vi "Arduino_FlowPump_Controller.vi"(0 "commands":refnum<queue>, 1 "GPIB ADDRESS":string(combo)="1", 2 "DECODER_DATA":refnum<queue>, 3 "measurements":refnum<queue>, 4 "Base Path":path=path "C:/Users/parad/Desktop/MAPI/last") -> ()   [LabVIEW 2021, in "GPIB_UART.lvlib"]
uses:
  GPIB_UART.lvlib
  startup_FSM.ctl
  dc_ps_FSM.ctl
  current_ramp_FSM.ctl
  Agilent_GPIB_FSM.vi
  Arduino_Serial_FSM.vi
  <vilib>/ErrorRing/Error Ring.xnode
panel:
  in  "START":i32
  in  "Next Current Ramp State":bool
  in  "Save As Button":bool
  in  "Stop Button":bool
  out "in_range":bool
  out "Output Current [mA]":i32 min=0 max=1 step=1
  in  "ADJUST":bool
  in  "Knob":ext(knob) scale=0.0..1.0
  out "Arduino UNO Controls":dbl[](graph)
  in  "VOLTAGE":bool
  in  "RESET & CLEAR":bool
  in  "READ ERROR":bool
  in  "Next":bool
  in  "CURRENT LIMIT [mA]":i32=700 min=0 max=1000 step=25
  in  "OUTPUT CHANNEL":enum32{"Channel 1", "Channel 2"}(radio)
  in  "STEP [mA]":i32=25 min=25 max=500 step=25
  in  "CURRENT RAMP":bool
  in  "POWER SUPPLY OUTPUT":bool
  in  "Read Button":bool
  out "SERIAL PORT":string(combo)="COM5"
  in  "Commands":string(combo)
  out "SAMPLE  COUNT":i32
  out "flow meas":dbl caption="FLOW RATE [SLPM]"
  in  "SAMP. FREQ. [HZ]":dbl=1.0 min=1.0 max=2.5 step=0.5
  in  "Clear Buffer":bool
  in  "Connect Button":bool
  out "BAUD":string="9600" caption="BAUD RATE (BIT/S)"
  # "POWER SUPPLY \nCONTROLS"
  # "OUTPUT CURRENT [A]"
  # "A"
  # "mA"
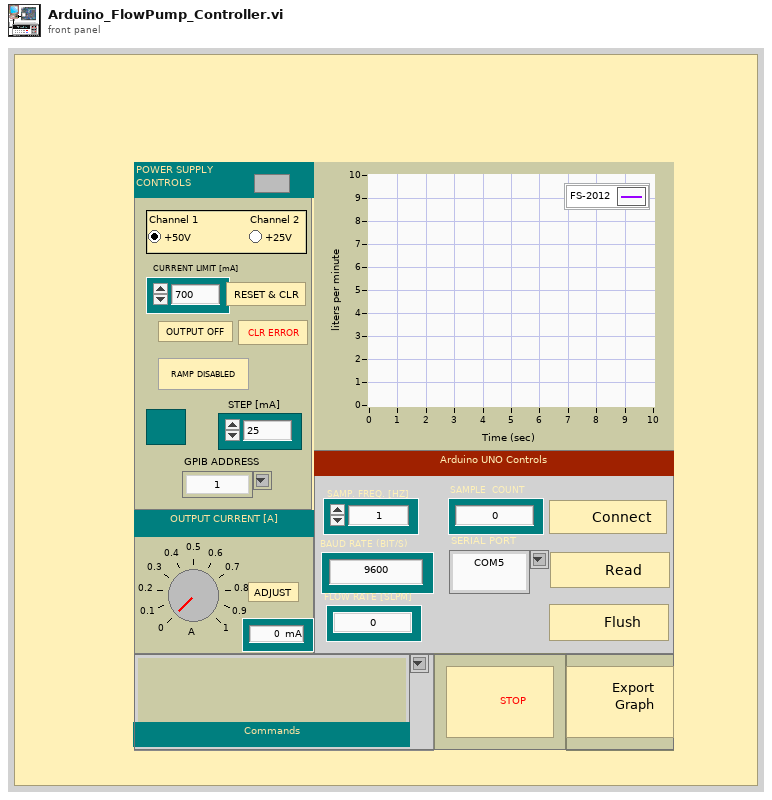
[diagram p1: front panel]
types:
  T1 = typedef "current_ramp_FSM.ctl" = enum16{"STATUS UPDATE", "SHUTDOWN", "INIT", "ERROR", "RAMP SETUP", "RAMP ENABLE", "RAMP DISABLE", "RAMP UP", "RAMP DOWN"}
  T2 = typedef "dc_ps_FSM.ctl" = enum16{"RESET", "SHUTDOWN", "VOLTAGE 12", "VOLTAGE 0", "INIT", "IDLE", "OUTPUT OFF", "OUTPUT ON", "OUT CURR", "SELECT CH", "LIMITS", "ENABLE RAMP", "RAMP UP", "RAMP DOWN", "RAMP STEP", "MEAS", "MEAS?", "ERROR", "READ ERROR", "DISABLE RAMP"}
  T3 = typedef "startup_FSM.ctl" = enum16{"SHUTDOWN", "IDLE", "INIT", "START MEAS", "READ", "STOP MEAS", "CHANGE BAUD", "CHANGE SAMP. FREQ.", "CHANGE PORT", "WRITE", "DISCONNECT", "CONNECT", "OUTPUT OFF", "MEAS_UNIT_L", "MEAS_UNIT_mL", "ERROR", "CLEAR BUFF", "OUTPUT ON"}
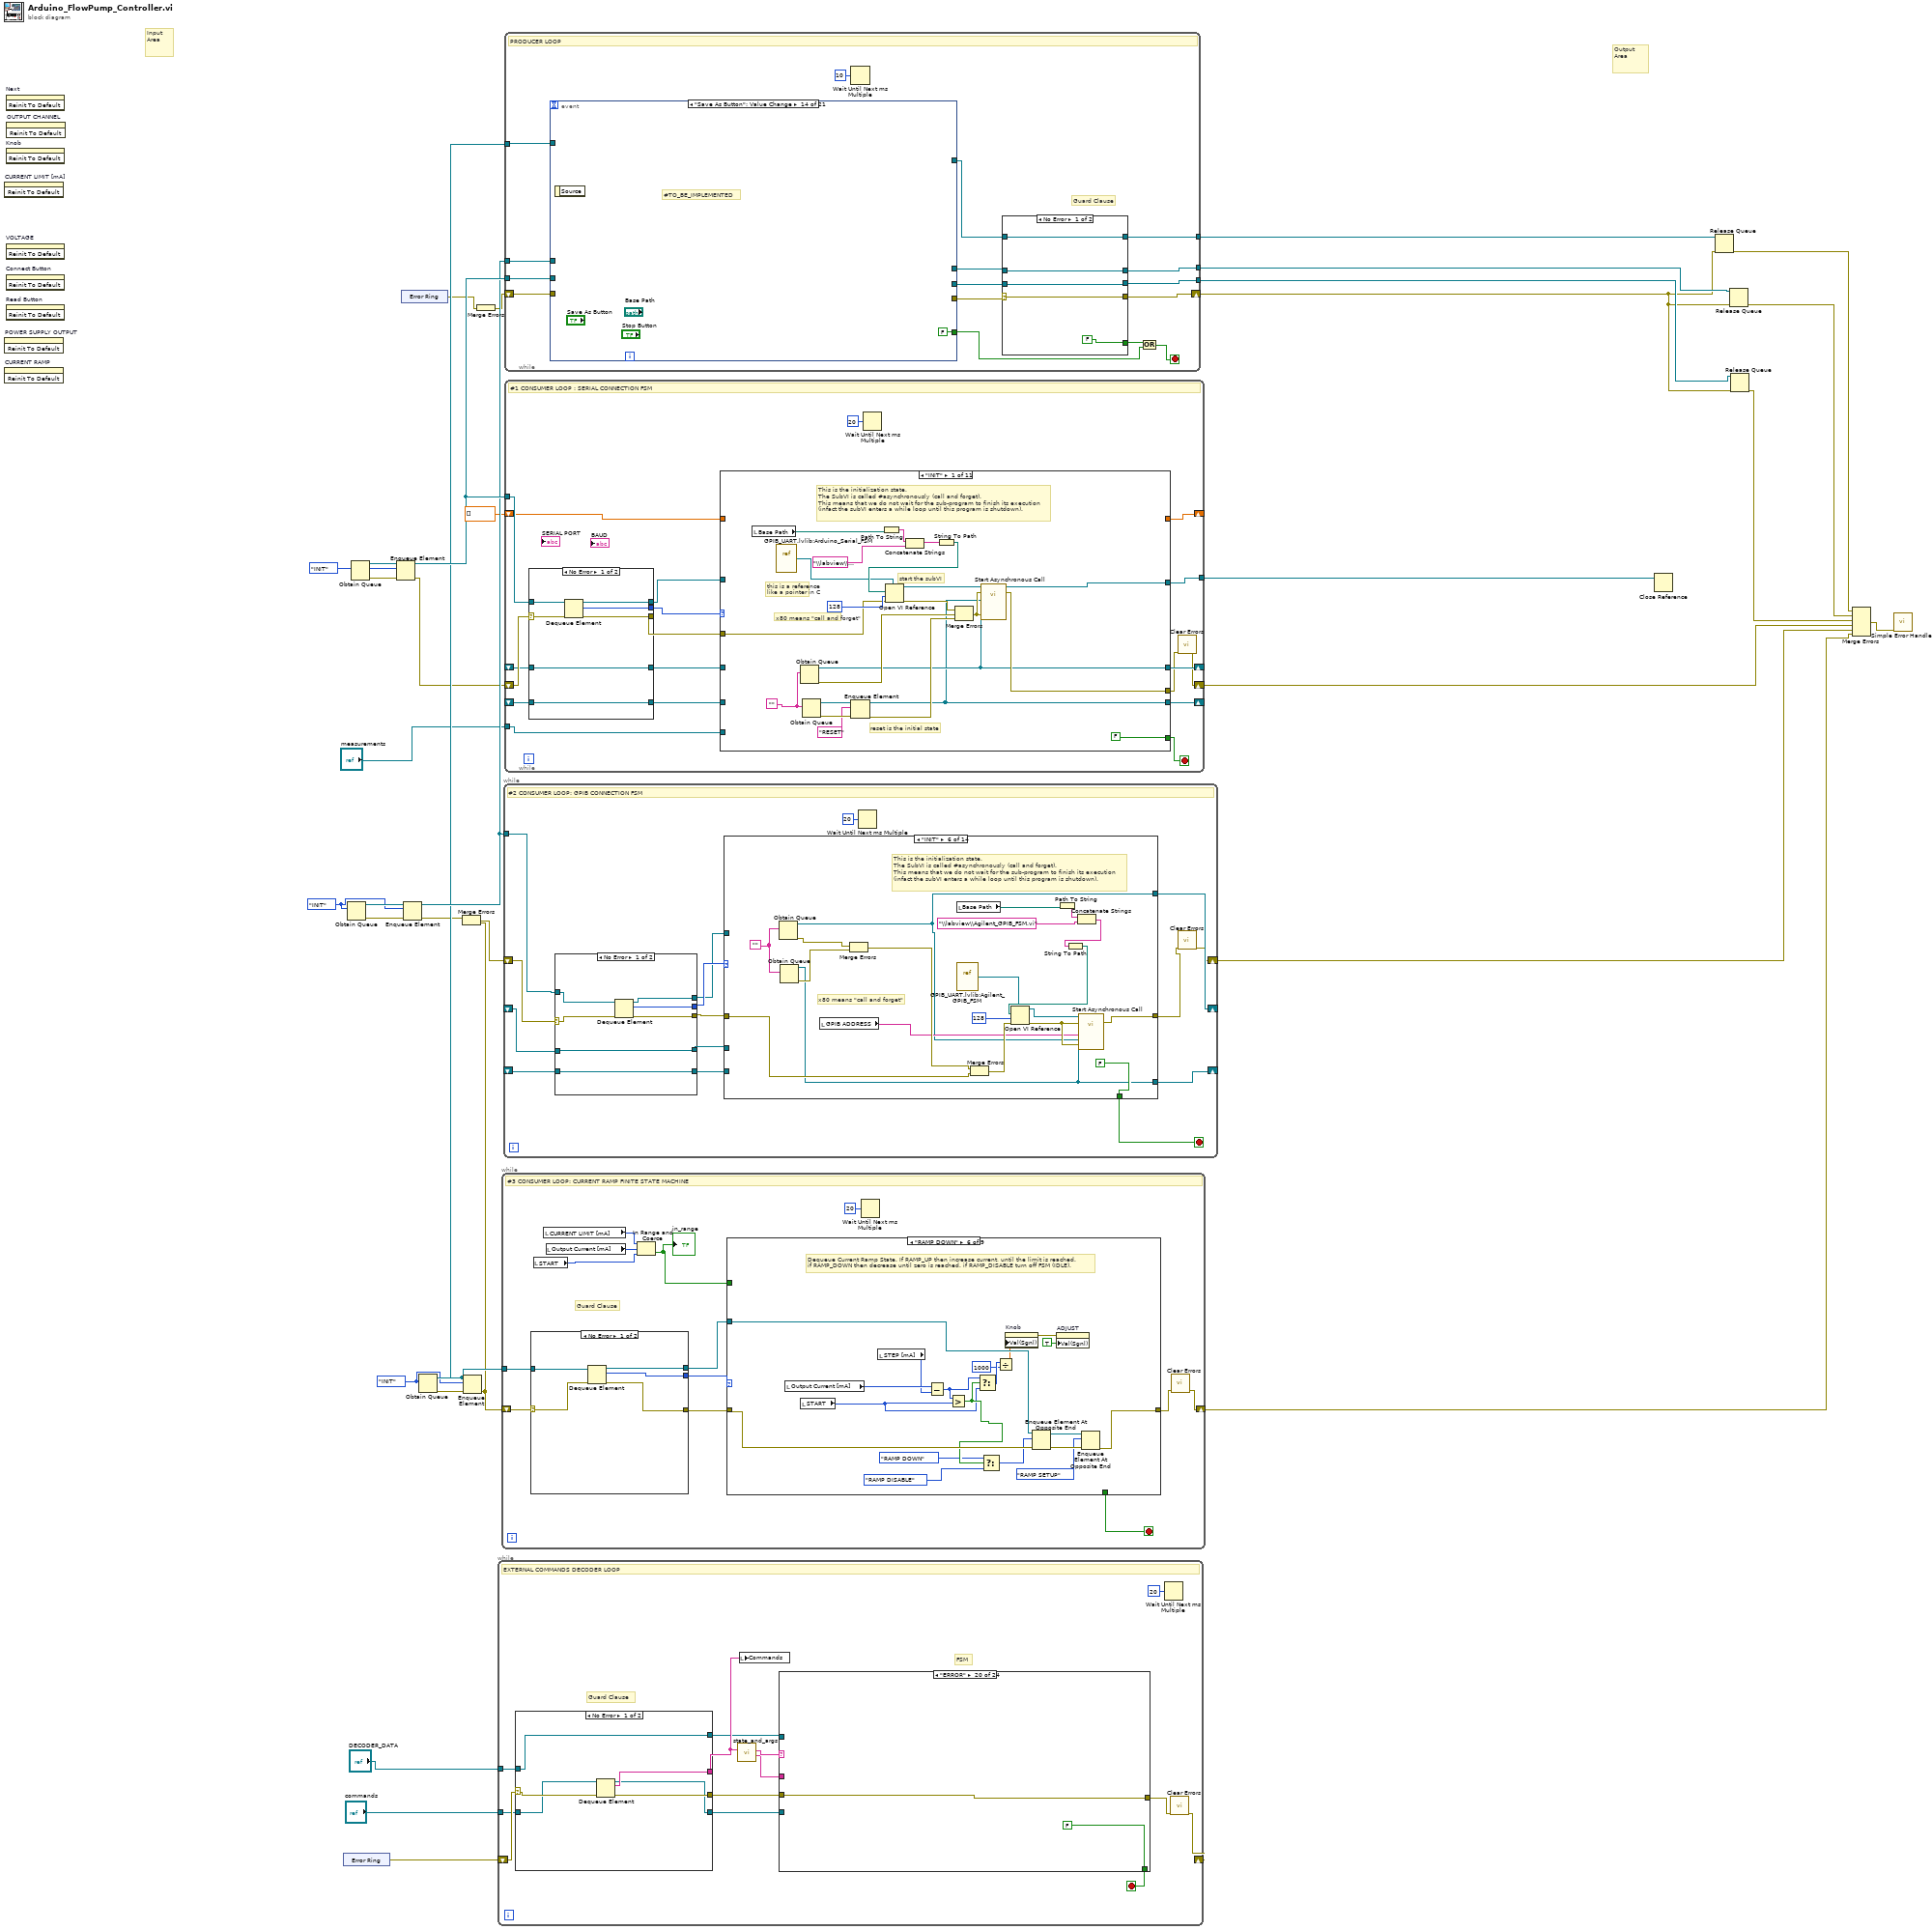
[diagram p0: block diagram]
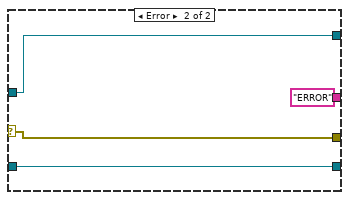
[diagram p2: hidden frame]
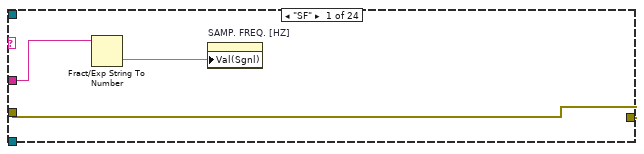
[diagram p3: hidden frame]
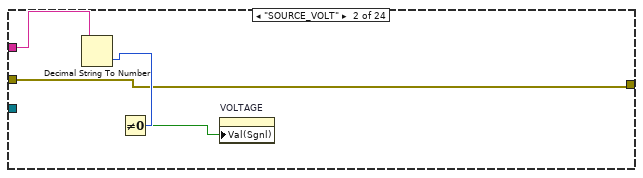
[diagram p4: hidden frame]
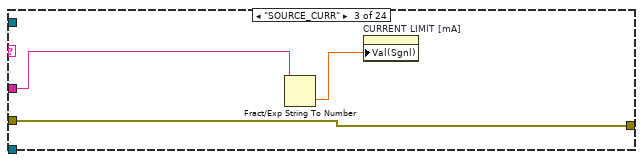
[diagram p5: hidden frame]
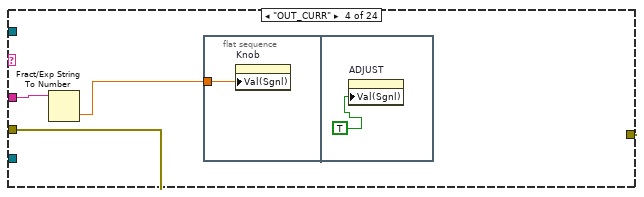
[diagram p6: hidden frame]
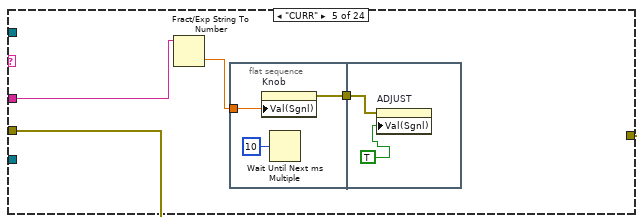
[diagram p7: hidden frame]
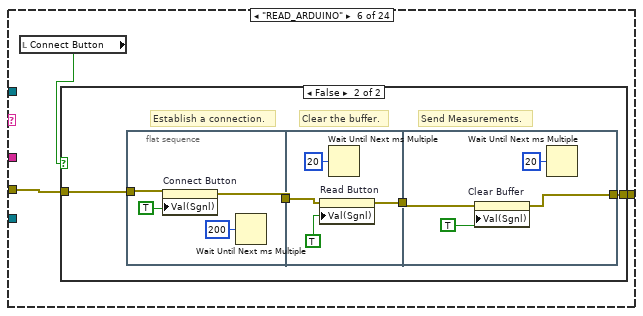
[diagram p8: hidden frame]
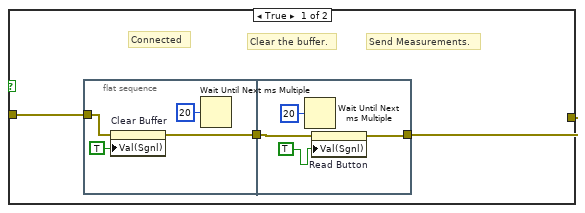
[diagram p9: hidden frame]
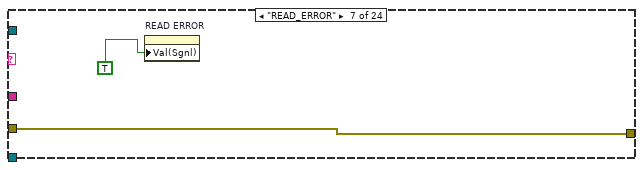
[diagram p10: hidden frame]
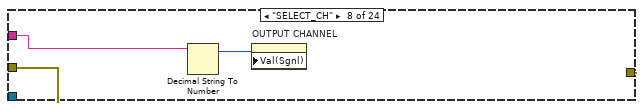
[diagram p11: hidden frame]
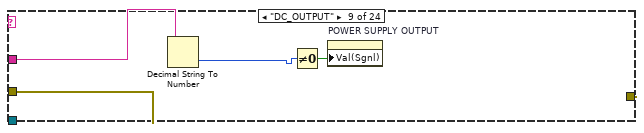
[diagram p12: hidden frame]
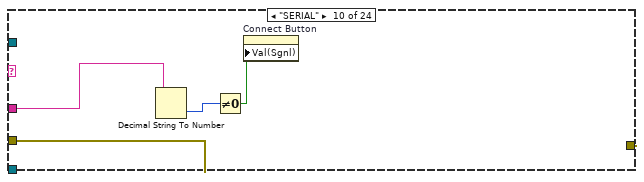
[diagram p13: hidden frame]
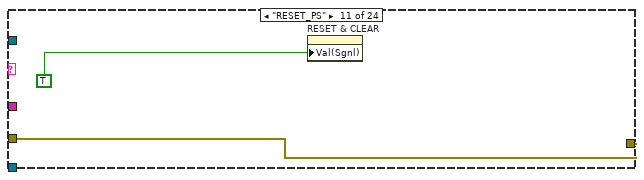
[diagram p14: hidden frame]
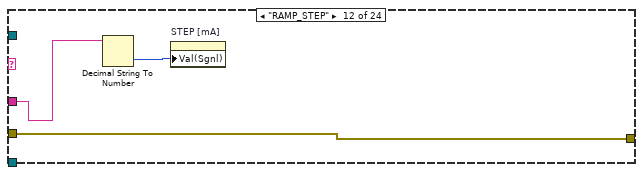
[diagram p15: hidden frame]
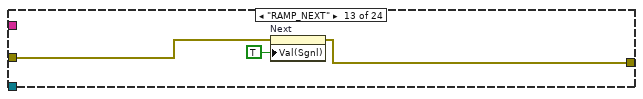
[diagram p16: hidden frame]
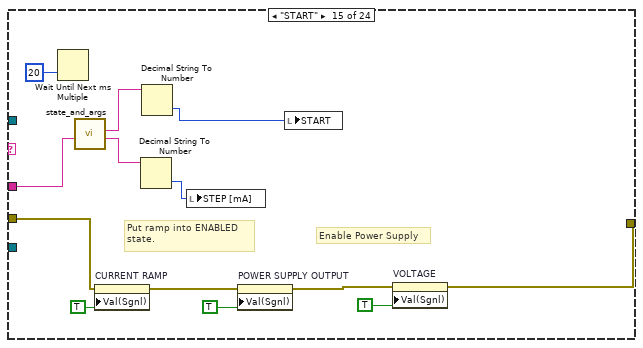
[diagram p18: hidden frame]
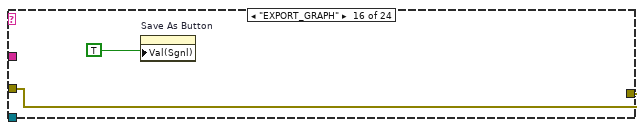
[diagram p19: hidden frame]
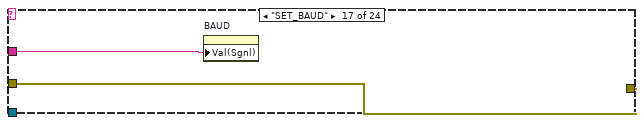
[diagram p20: hidden frame]
diagram:
  w14 = current_ramp_FSM."INIT" ("Enum")
  w29 = dc_ps_FSM."INIT" ("DC Power Supply FSM")
  w30 = startup_FSM."INIT" ("element")
  # "Output\nArea"
  # "Input\nArea"
  n1 = invoke on="CURRENT LIMIT [mA]" class="DigNum (strict)" method="Reinit To Default"() -> ()  [unwired: 3 in, 3 out]
  n2 = invoke on="POWER SUPPLY OUTPUT" class="Bool (strict)" method="Reinit To Default"() -> ()  [unwired: 3 in, 3 out]
  n3 = invoke on="CURRENT RAMP" class="Bool (strict)" method="Reinit To Default"() -> ()  [unwired: 3 in, 3 out]
  n4 = invoke on="Next" class="Bool (strict)" method="Reinit To Default"() -> ()  [unwired: 3 in, 3 out]
  n5 = invoke on="Knob" class="Knob (strict)" method="Reinit To Default"() -> ()  [unwired: 3 in, 3 out]
  n6 = invoke on="VOLTAGE" class="Bool (strict)" method="Reinit To Default"() -> ()  [unwired: 3 in, 3 out]
  n7 = invoke on="Connect Button" class="Bool (strict)" method="Reinit To Default"() -> ()  [unwired: 3 in, 3 out]
  n8 = invoke on="Read Button" class="Bool (strict)" method="Reinit To Default"() -> ()  [unwired: 3 in, 3 out]
  n9 = invoke on="OUTPUT CHANNEL" class="RadioBtnsControl (strict)" method="Reinit To Default"() -> ()  [unwired: 3 in, 3 out]
  n10 = xnode "Error Ring"() -> ("error out"=w15:errorcluster)
  n11 = Obtain Queue(element data type=w29) -> (queue out=w32:refnum<queue>, error out=w31:errorcluster)  [unwired: 4 in, 1 out]
  n12 = Obtain Queue(element data type=w30) -> (queue out=w35:refnum<queue>, error out=w34:errorcluster)  [unwired: 4 in, 1 out]
  n13 = Enqueue Element(queue=w35, element=w30, error in (no error)=w34) -> (queue out=w33:refnum<queue>, error out=w7:errorcluster)  [unwired: 1 in, 1 out]
  n14 = xnode "Error Ring"() -> ("error out"=w11:errorcluster)
  n15 = Enqueue Element(queue=w32, element=w29, error in (no error)=w31) -> (queue out=w28:refnum<queue>, error out=w9:errorcluster)  [unwired: 1 in, 1 out]
  n16 = Obtain Queue(element data type=w14) -> (queue out=w19:refnum<queue>, error out=w18:errorcluster)  [unwired: 4 in, 1 out]
  n17 = Enqueue Element(queue=w19, element=w14, error in (no error)=w18) -> (queue out=w17:refnum<queue>, error out=w8:errorcluster)  [unwired: 1 in, 1 out]
  n18 = Merge Errors(w9, w8) -> (w10:errorcluster)
  n19 = Merge Errors(w11) -> (w12:errorcluster)
  n20 = while {
    shift-right: [w37] -> _
    shift-left: w15 -> [w47]
    tunnel: "commands" -> [w44]
    tunnel: "DECODER_DATA" -> [w39]
    stop <- w45 stop-if-true
    # "FSM"
    # "Guard Clause"
    # "EXTERNAL COMMANDS DECODER LOOP"
    n21 = case shown="No Error" w47 {
      selector: w47 -> [w54 w56]
      tunnel: [w53 "ERROR" ("element")] -> w40
      tunnel: [w52 w56] -> w46
      tunnel: [w49 w57] -> w43
      tunnel: w44 -> [w51 w57]
      tunnel: w39 -> [w50 w55]
      tunnel: [w50 w55] -> w38
      frame No Error {
        n22 = Dequeue Element(queue=w51, error in (no error)=w54) -> (queue out=w49:refnum<queue>, element=w53:string, error out=w52:errorcluster)  [unwired: 1 in, 1 out]
      }
      frame Error {
      }
    }
    n23 = call "state_and_args.vi"("String"=w40) -> ("Arguments"=w41:string, "State"=w42:string)  [unwired: 9 in]
    n24 = local write "Commands"(w40) -> ()
    n25 = case shown="\"ERROR\"" w42 {
      tunnel: w46 -> [w59 w62 w66 w70 w76 w85 w113 w115 w118 w122 w126 w128 w131 w134 w144 w148 w150 w152 w157 w161 w163 w170 w179 w182]
      tunnel: [_ _ _ _ _ _ _ _ _ _ _ _ _ _ _ _ _ _ _ FALSE FALSE _ TRUE _] -> w45
      tunnel: w43 -> [_ _ _ _ _ _ _ _ _ _ _ _ _ _ _ _ _ _ _ _ _ _ _ _]
      tunnel: [w59 w62 w66 w70 w76 w84 w113 w115 w118 w122 w126 w128 w132 w134 w141 w148 w150 w152 w156 w161 w163 w166 w180 w182] -> w36
      tunnel: w41 -> [w60 w63 w67 w69 w75 _ _ w116 w119 w123 _ w129 _ _ w140 _ w151 w153 _ _ _ w169 _ _]
      tunnel: w38 -> [_ _ _ _ _ _ _ _ _ _ _ _ _ _ _ _ _ _ w160 _ _ _ _ _]
      frame "SF" {
        n26 = Fract/Exp String To Number(string=w60) -> (number=w61:dbl)  [unwired: 3 in, 1 out]
        n27 = property on="SAMP. FREQ. [HZ]" class="DigNum (strict)"("Val(Sgnl)"=w61) -> ()  [unwired: 2 in, 2 out]
      }
      frame "SOURCE_VOLT" {
        n28 = Decimal String To Number(string=w63) -> (number=w65:i32)  [unwired: 2 in, 1 out]
        n29 = Not Equal To 0?(x=w65) -> (x != 0?=w64:bool)
        n30 = property on="VOLTAGE" class="Bool (strict)"("Val(Sgnl)"=w64) -> ()  [unwired: 2 in, 2 out]
      }
      frame "SOURCE_CURR" {
        n31 = Fract/Exp String To Number(string=w67) -> (number=w68:dbl)  [unwired: 3 in, 1 out]
        n32 = property on="CURRENT LIMIT [mA]" class="DigNum (strict)"("Val(Sgnl)"=w68) -> ()  [unwired: 2 in, 2 out]
      }
      frame "OUT_CURR" {
        n33 = Fract/Exp String To Number(string=w69) -> (number=w71:dbl)  [unwired: 3 in, 1 out]
        n34 = flat-sequence {
          tunnel: w71 -> [w72]
          frame #0 {
            n35 = property on="Knob" class="Knob (strict)"("Val(Sgnl)"=w72) -> ()  [unwired: 2 in, 2 out]
          }
          frame #1 {
            n36 = property on="ADJUST" class="Bool (strict)"("Val(Sgnl)"=TRUE) -> ()  [unwired: 2 in, 2 out]
          }
        }
      }
      frame "CURR" {
        n37 = Fract/Exp String To Number(string=w75) -> (number=w77:dbl)  [unwired: 3 in, 1 out]
        n38 = flat-sequence {
          tunnel: w77 -> [w80]
          tunnel: [w78] -> w74
          tunnel: w74 -> [w81]
          frame #0 {
            n39 = property on="Knob" class="Knob (strict)"("Val(Sgnl)"=w80) -> (error out=w78:errorcluster)  [unwired: 2 in, 1 out]
            n40 = Wait Until Next ms Multiple(millisecond multiple=u32 10) -> ()  [unwired: 1 out]
          }
          frame #1 {
            n41 = property on="ADJUST" class="Bool (strict)"(error in=w81, "Val(Sgnl)"=TRUE) -> ()  [unwired: 1 in, 2 out]
          }
        }
      }
      frame "READ_ARDUINO" {
        n42 = local read "Connect Button"() -> (w83:bool)
        n43 = case shown="False" w83 {
          tunnel: w85 -> [w86 w100]
          tunnel: [w88 w97] -> w84
          frame True {
            # "Send Measurements."
            # "Clear the buffer."
            # "Connected"
            n44 = flat-sequence {
              tunnel: [w90] -> w87
              tunnel: w86 -> [w91]
              tunnel: [w95] -> w88
              tunnel: w87 -> [w94]
              frame #0 {
                n45 = property on="Clear Buffer" class="Bool (strict)"(error in=w91, "Val(Sgnl)"=TRUE ("Value (Signaling)")) -> (error out=w90:errorcluster)  [unwired: 1 in, 1 out]
                n46 = Wait Until Next ms Multiple(millisecond multiple=u32 20) -> ()  [unwired: 1 out]
              }
              frame #1 {
                n47 = Wait Until Next ms Multiple(millisecond multiple=u32 20) -> ()  [unwired: 1 out]
                n48 = property on="Read Button" class="Bool (strict)"(error in=w94, "Val(Sgnl)"=TRUE ("Value (Signaling)")) -> (error out=w95:errorcluster)  [unwired: 1 in, 1 out]
              }
            }
          }
          frame False {
            # "Send Measurements."
            # "Clear the buffer."
            # "Establish a connection."
            n49 = flat-sequence {
              tunnel: w100 -> [w103]
              tunnel: [w102] -> w99
              tunnel: w99 -> [w107]
              tunnel: [w106] -> w98
              tunnel: w98 -> [w110]
              tunnel: [w109] -> w97
              frame #0 {
                n50 = property on="Connect Button" class="Bool (strict)"(error in=w103, "Val(Sgnl)"=TRUE ("Value (Signaling)")) -> (error out=w102:errorcluster)  [unwired: 1 in, 1 out]
                n51 = Wait Until Next ms Multiple(millisecond multiple=u32 200) -> ()  [unwired: 1 out]
              }
              frame #1 {
                n52 = property on="Read Button" class="Bool (strict)"(error in=w107, "Val(Sgnl)"=TRUE ("Value (Signaling)")) -> (error out=w106:errorcluster)  [unwired: 1 in, 1 out]
                n53 = Wait Until Next ms Multiple(millisecond multiple=u32 20) -> ()  [unwired: 1 out]
              }
              frame #2 {
                n54 = property on="Clear Buffer" class="Bool (strict)"(error in=w110, "Val(Sgnl)"=TRUE ("Value (Signaling)")) -> (error out=w109:errorcluster)  [unwired: 1 in, 1 out]
                n55 = Wait Until Next ms Multiple(millisecond multiple=u32 20) -> ()  [unwired: 1 out]
              }
            }
          }
        }
      }
      frame "READ_ERROR" {
        n56 = property on="READ ERROR" class="Bool (strict)"("Val(Sgnl)"=TRUE) -> ()  [unwired: 2 in, 2 out]
      }
      frame "SELECT_CH" {
        n57 = Decimal String To Number(string=w116) -> (offset past number=w117:i32)  [unwired: 2 in, 1 out]
        n58 = property on="OUTPUT CHANNEL" class="RadioBtnsControl (strict)"("Val(Sgnl)"=w117) -> ()  [unwired: 2 in, 2 out]
      }
      frame "DC_OUTPUT" {
        n59 = Decimal String To Number(string=w119) -> (number=w121:i32)  [unwired: 2 in, 1 out]
        n60 = Not Equal To 0?(x=w121) -> (x != 0?=w120:bool)
        n61 = property on="POWER SUPPLY OUTPUT" class="Bool (strict)"("Val(Sgnl)"=w120) -> ()  [unwired: 2 in, 2 out]
      }
      frame "SERIAL" {
        n62 = Decimal String To Number(string=w123) -> (number=w124:i32)  [unwired: 2 in, 1 out]
        n63 = Not Equal To 0?(x=w124) -> (x != 0?=w125:bool)
        n64 = property on="Connect Button" class="Bool (strict)"("Val(Sgnl)"=w125) -> ()  [unwired: 2 in, 2 out]
      }
      frame "RESET_PS" {
        n65 = property on="RESET & CLEAR" class="Bool"("Val(Sgnl)"=TRUE) -> ()  [unwired: 2 in, 2 out]
      }
      frame "RAMP_STEP" {
        n66 = Decimal String To Number(string=w129) -> (number=w130:i32)  [unwired: 2 in, 1 out]
        n67 = property on="STEP [mA]" class="DigNum (strict)"("Val(Sgnl)"=w130) -> ()  [unwired: 2 in, 2 out]
      }
      frame "RAMP_NEXT" {
        n68 = property on="Next" class="Bool (strict)"(error in=w131, "Val(Sgnl)"=TRUE ("Value (Signaling)")) -> (error out=w132:errorcluster)  [unwired: 1 in, 1 out]
      }
      frame "RAMP_ENABLE" {
      }
      frame "START" {
        # "Enable Power Supply"
        # "Put ramp into ENABLED\nstate."
        n69 = Wait Until Next ms Multiple(millisecond multiple=u32 20) -> ()  [unwired: 1 out]
        n70 = call "state_and_args.vi"("String"=w140) -> ("Arguments"=w137:string, "State"=w138:string)  [unwired: 9 in]
        n71 = property on="CURRENT RAMP" class="Bool (strict)"(error in=w144, "Val(Sgnl)"=TRUE ("Value (Signaling)")) -> (error out=w143:errorcluster)  [unwired: 1 in, 1 out]
        n72 = Decimal String To Number(string=w137) -> (number=w136:i32)  [unwired: 2 in, 1 out]
        n73 = Decimal String To Number(string=w138) -> (number=w139:i32)  [unwired: 2 in, 1 out]
        n74 = local write "STEP [mA]"(w136) -> ()
        n75 = property on="POWER SUPPLY OUTPUT" class="Bool (strict)"(error in=w143, "Val(Sgnl)"=TRUE ("Value (Signaling)")) -> (error out=w142:errorcluster)  [unwired: 1 in, 1 out]
        n76 = local write "START"(w139) -> ()
        n77 = property on="VOLTAGE" class="Bool (strict)"(error in=w142, "Val(Sgnl)"=TRUE ("Value (Signaling)")) -> (error out=w141:errorcluster)  [unwired: 1 in, 1 out]
      }
      frame "EXPORT_GRAPH" {
        n78 = property on="Save As Button" class="Bool (strict)"("Val(Sgnl)"=TRUE ("Value (Signaling)")) -> ()  [unwired: 2 in, 2 out]
      }
      frame "SET_BAUD" {
        n79 = property on="BAUD" class="Str"("Val(Sgnl)"=w151) -> ()  [unwired: 2 in, 2 out]
      }
      frame "READ_ALL" {
        n80 = Decimal String To Number(string=w153) -> (number=w154:i32)  [unwired: 2 in, 1 out]
        n81 = Not Equal To 0?(x=w154) -> (x != 0?=w155:bool)
        n82 = property on="Read Button" class="Bool (strict)"("Val(Sgnl)"=w155) -> ()  [unwired: 2 in, 2 out]
      }
      frame "CURR?" {
        n83 = local read "Output Current [mA]"() -> (w159:i32)
        n84 = Number To Decimal String(number=w159) -> (decimal integer string=w158:string)  [unwired: 1 in]
        n85 = Enqueue Element(queue=w160, element=w158, error in (no error)=w157) -> (error out=w156:errorcluster)  [unwired: 1 in, 2 out]
      }
      frame "ERROR" {
      }
      frame "CLEAR_BUFF" {
        n86 = property on="Clear Buffer" class="Bool (strict)"("Val(Sgnl)"=TRUE ("Value (Signaling)")) -> ()  [unwired: 2 in, 2 out]
      }
      frame "SET_PORT" {
        n87 = local read "Connect Button"() -> (w171:bool)
        n88 = case shown="False" w171 {
          tunnel: w170 -> [w172 w176]
          tunnel: [w172 w175] -> w167
          tunnel: [w173 w174] -> w168
          tunnel: w169 -> [w173 w174]
          frame False {
          }
          frame True {
            n89 = property on="Connect Button" class="Bool (strict)"(error in=w176, "Val(Sgnl)"=FALSE ("Value (Signaling)")) -> (error out=w175:errorcluster)  [unwired: 1 in, 1 out]
          }
        }
        n90 = property on="SERIAL PORT" class="CmbBox"(error in=w167, "Val(Sgnl)"=w168) -> (error out=w166:errorcluster)  [unwired: 1 in, 1 out]
      }
      frame "SHUTDOWN" {
        n91 = property on="Stop Button" class="Bool (strict)"(error in=w179, "Val(Sgnl)"=TRUE) -> (error out=w180:errorcluster)  [unwired: 1 in, 1 out]
      }
      frame "Def", Default {
        # "default: do nothing"
      }
    }
    n92 = Wait Until Next ms Multiple(millisecond multiple=u32 20 ("milliseconds to wait")) -> ()  [unwired: 1 out]
    n93 = call <vilib>:"Clear Errors.vi"("error in (no error)"=w36) -> ("error out"=w37:errorcluster)  [unwired: 5 in, 1 out]
  }
  n94 = while {
    shift-right: [w184] -> w13
    shift-left: w8 -> [w193]
    tunnel: w17 -> [w194]
    stop <- w190 stop-if-true
    # "Guard Clause"
    # "#3 CONSUMER LOOP: CURRENT RAMP FINITE STATE MACHINE"
    n95 = case shown="No Error" w193 {
      selector: w193 -> [w262 w265]
      tunnel: w194 -> [w263 w266]
      tunnel: [w261 w265] -> w192
      tunnel: [w260 w266] -> w191
      tunnel: [w259 current_ramp_FSM."ERROR" ("Enum")] -> w189
      frame No Error {
        n96 = Dequeue Element(queue=w263, error in (no error)=w262) -> (queue out=w260:refnum<queue>, element=w259:T1, error out=w261:errorcluster)  [unwired: 1 in, 1 out]
      }
      frame Error {
      }
    }
    n97 = local read "START"() -> (w183:i32)
    n98 = local read "CURRENT LIMIT [mA]"() -> (w188:i32)
    n99 = local read "Output Current [mA]"() -> (w187:i32)
    n100 = In Range and Coerce(upper limit=w188, x=w187, lower limit=w183) -> (In Range?=w186:bool)  [unwired: 1 out]
    "in_range" <- w186
    n101 = case shown="\"RAMP DOWN\"" w189 {
      tunnel: w192 -> [w199 w202 w210 w211 w214 w234 w254 w258 _]
      tunnel: [w196 w202 w209 w211 w213 w223 w239 w257 _] -> w185
      tunnel: w191 -> [w200 _ w208 _ _ w227 w246 w255 _]
      tunnel: [TRUE FALSE _ _ _ _ _ FALSE _] -> w190
      tunnel: w186 -> [_ _ _ _ _ _ w238 _ _]
      frame "SHUTDOWN" {
        n102 = Preview Queue Element(queue=w200, error in (no error)=w199) -> (queue out=w198:refnum<queue>, error out=w197:errorcluster)  [unwired: 1 in, 2 out]
        n103 = Preview Queue Element(queue=w198, error in (no error)=w197) -> (error out=w196:errorcluster)  [unwired: 1 in, 3 out]
      }
      frame "INIT", Default {
      }
      frame "RAMP ENABLE" {
        n104 = local read "STEP [mA]"() -> (w205:i32)
        n105 = Subtract(x="START", y=w205) -> (x-y=w204:i32)
        n106 = local write "Output Current [mA]"(w204) -> ()
        n107 = Enqueue Element(queue=w208, element=current_ramp_FSM."RAMP UP", error in (no error)=w210) -> (error out=w209:errorcluster)  [unwired: 1 in, 2 out]
      }
      frame "RAMP DISABLE" {
        n108 = property on="CURRENT RAMP" class="Bool (strict)"("Val(Sgnl)"=FALSE ("Value (Signaling)")) -> ()  [unwired: 2 in, 2 out]
      }
      frame "RAMP SETUP" {
        # "IDLE STATE"
        n109 = event shown="[0] \"Next Current Ramp State\": Value Change" {
          selector: _ -> [_]
          dyn-events: _ -> [_]
          timeout: _ -> [_]
          tunnel: [w215] -> w213
          tunnel: w214 -> [w215]
          event "Next Current Ramp State": Value Change {
            n110 = event-data() -> ()  [unwired: 1 in, 1 out]
          }
        }
      }
      frame "RAMP DOWN" {
        # "Dequeue Current Ramp State. If RAMP_UP then increase current, until the limit is reached.\nif RAMP_DOWN then decrease until zero is reached. if RAMP_DISABLE turn off FSM (IDLE)."
        n111 = local read "Output Current [mA]"() -> (w233:i32)
        n112 = local read "START"() -> (w219:i32)
        n113 = local read "STEP [mA]"() -> (w232:i32)
        n114 = Subtract(x=w233, y=w232) -> (x-y=w231:i32)
        n115 = Greater?(x=w231, y=w219) -> (0:w228:bool)
        n116 = Select(t=w231, s=w228, f=w219) -> (s? t:f=w218:i32)
        n117 = Select(t=current_ramp_FSM."RAMP DOWN" ("element"), s=w228, f=current_ramp_FSM."RAMP DISABLE") -> (s? t:f=w226:T1)
        n118 = Divide(x=w218, y=1000) -> (x/y=w216:dbl)
        n119 = property on="Knob" class="Knob (strict)"("Val(Sgnl)"=w216) -> (error out=w230:errorcluster)  [unwired: 2 in, 1 out]
        n120 = Enqueue Element At Opposite End(queue=w227, element=w226, error in (no error)=w234) -> (queue out=w222:refnum<queue>, error out=w221:errorcluster)  [unwired: 1 in, 1 out]
        n121 = property on="ADJUST" class="Bool (strict)"(error in=w230, "Val(Sgnl)"=TRUE ("Value (Signaling)")) -> ()  [unwired: 1 in, 2 out]
        n122 = Enqueue Element At Opposite End(queue=w222, element=current_ramp_FSM."RAMP SETUP", error in (no error)=w221) -> (error out=w223:errorcluster)  [unwired: 1 in, 2 out]
      }
      frame "RAMP UP" {
        # "Dequeue Current Ramp State. If RAMP_UP then increase current, until the limit is reached."
        n123 = local read "Output Current [mA]"() -> (w253:i32)
        n124 = local read "CURRENT LIMIT [mA]"() -> (w249:i32)
        n125 = local read "STEP [mA]"() -> (w252:i32)
        n126 = Add(x=w253, y=w252) -> (x+y=w250:i32)
        n127 = Less?(x=w250, y=w249) -> (x < y?=w251:bool)
        n128 = Select(t=w250, s=w251, f=w249) -> (s? t:f=w237:i32)
        n129 = Select(t=current_ramp_FSM."RAMP UP" ("element"), s=w238, f=current_ramp_FSM."RAMP DOWN") -> (s? t:f=w243:T1)
        n130 = Divide(x=w237, y=1000) -> (x/y=w235:dbl)
        n131 = property on="Knob" class="Knob (strict)"("Val(Sgnl)"=w235) -> (error out=w248:errorcluster)  [unwired: 2 in, 1 out]
        n132 = Enqueue Element At Opposite End(queue=w246, element=w243, error in (no error)=w254) -> (queue out=w242:refnum<queue>, error out=w241:errorcluster)  [unwired: 1 in, 1 out]
        n133 = Enqueue Element At Opposite End(queue=w242, element=current_ramp_FSM."RAMP SETUP", error in (no error)=w241) -> (error out=w239:errorcluster)  [unwired: 1 in, 2 out]
        n134 = property on="ADJUST" class="Bool (strict)"(error in=w248, "Val(Sgnl)"=TRUE ("Value (Signaling)")) -> ()  [unwired: 1 in, 2 out]
      }
      frame "ERROR" {
        n135 = Preview Queue Element(queue=w255, error in (no error)=w258) -> (error out=w257:errorcluster)  [unwired: 1 in, 3 out]
      }
      frame "STATUS UPDATE" {
      }
    }
    n136 = Wait Until Next ms Multiple(millisecond multiple=u32 20) -> ()  [unwired: 1 out]
    n137 = call <vilib>:"Clear Errors.vi"("error in (no error)"=w185) -> ("error out"=w184:errorcluster)  [unwired: 5 in, 1 out]
  }
  n138 = while {
    tunnel: w28 -> [w280]
    shift-right: [w268] -> w22
    shift-left: w10 -> [w281]
    shift-right: [w271] -> _
    shift-left: _ -> [w270]
    shift-right: [w272] -> _
    shift-left: _ -> [w273]
    stop <- w276 stop-if-true
    # "#2 CONSUMER LOOP: GPIB CONNECTION FSM"
    n139 = case shown="No Error" w281 {
      selector: w281 -> [w418 w422]
      tunnel: w280 -> [w419 w423]
      tunnel: [w417 dc_ps_FSM."ERROR" ("DC Power Supply FSM")] -> w279
      tunnel: [w416 w423] -> w278
      tunnel: [w415 w422] -> w277
      tunnel: w273 -> [w414 w420]
      tunnel: [w414 w420] -> w274
      tunnel: [w413 w421] -> w269
      tunnel: w270 -> [w413 w421]
      frame No Error {
        n140 = Dequeue Element(queue=w419, error in (no error)=w418) -> (queue out=w416:refnum<queue>, element=w417:T2, error out=w415:errorcluster)  [unwired: 1 in, 1 out]
      }
      frame Error {
      }
    }
    n141 = case shown="\"INIT\"" w279 {
      tunnel: w278 -> [_ _ _ _ _ _ w354 _ _ _ _ _ _ _]
      tunnel: w277 -> [w286 w293 w304 w309 w332 w340 w353 w378 w385 w391 w396 w403 w408 w412]
      tunnel: [w285 w291 w299 w308 w327 w350 w355 w380 w385 w389 w395 w402 w407 w412] -> w267
      tunnel: w274 -> [w282 w288 w296 w305 w324 _ w359 w377 w384 w387 w394 w399 w404 w410]
      tunnel: [_ _ _ _ _ FALSE TRUE FALSE _ _ _ _ _ _] -> w276
      tunnel: [w282 w288 w296 w305 w324 w333 w359 w375 w384 w387 w394 w399 w404 w410] -> w272
      tunnel: [w283 w289 w295 w306 w325 w334 w356 w374 w383 w386 w392 w398 w405 w411] -> w271
      tunnel: w269 -> [w284 w290 w297 w307 w326 _ w360 w376 w383 w388 w393 w400 w406 w411]
      frame "OUTPUT OFF" {
        # "Sends a command to the Finite State Machine to turn off its output"
        n142 = Enqueue Element(queue=w284, element="OUTPUT OFF", error in (no error)=w286) -> (queue out=w283:refnum<queue>, error out=w285:errorcluster)  [unwired: 1 in, 1 out]
      }
      frame "OUTPUT ON" {
        # "Sends a command to the Finite State Machine to turn off its output"
        n143 = Enqueue Element(queue=w290, element="OUTPUT ON", error in (no error)=w293) -> (queue out=w289:refnum<queue>, error out=w291:errorcluster)  [unwired: 1 in, 1 out]
      }
      frame "OUT CURR" {
        # "Sends a command to the Finite State Machine to change the output current"
        n144 = local read "Knob"() -> (w294:ext)
        n145 = Number To Fractional String(use system decimal point (T)=FALSE, number=w294, precision (6)=i16 4) -> (F-format string=w303:string)  [unwired: 1 in]
        n146 = Concatenate Strings("CURR " ("element"), w303) -> (w300:string)
        n147 = Enqueue Element(queue=w297, element=w300, error in (no error)=w304) -> (queue out=w295:refnum<queue>, error out=w299:errorcluster)  [unwired: 1 in, 1 out]
      }
      frame "SELECT CH" {
        # "Sends a command to the Finite State Machine to change the output Channel (either 25 or 50V)"
        n148 = case shown="\"Channel 2\", Default" "OUTPUT CHANNEL" {
          tunnel: w309 -> [w315 w320]
          tunnel: [w313 w318] -> w308
          tunnel: w307 -> [w312 w316]
          tunnel: [w311 w317] -> w306
          frame "Channel 1" {
            n149 = Enqueue Element(queue=w312, element="VOLT:RANG P50V", error in (no error)=w315) -> (queue out=w311:refnum<queue>, error out=w313:errorcluster)  [unwired: 1 in, 1 out]
          }
          frame "Channel 2", Default {
            n150 = Enqueue Element(queue=w316, element="VOLT:RANG P25V", error in (no error)=w320) -> (queue out=w317:refnum<queue>, error out=w318:errorcluster)  [unwired: 1 in, 1 out]
          }
        }
      }
      frame "LIMITS" {
        # "Sends a command to the Finite State Machine to change the current limit"
        n151 = Divide(x="CURRENT LIMIT [mA]", y=1000.0) -> (x/y=w321:dbl)
        n152 = Number To Fractional String(number=w321, precision (6)=i16 4) -> (F-format string=w329:string)  [unwired: 2 in]
        n153 = Concatenate Strings("CURR:PROT " ("element"), w329) -> (w331:string)
        n154 = Enqueue Element(queue=w326, element=w331, error in (no error)=w332) -> (queue out=w325:refnum<queue>, error out=w327:errorcluster)  [unwired: 1 in, 1 out]
      }
      frame "INIT" {
        w344 = ""
        # "x80 means \"call and forget\""
        # "This is the initialization state.\nThe SubVI is called #asynchronously (call and forget).\nThis means that we do not wait for the sub-program to finish its execution\n(infact the subVI enters a while loop until this program is shutdown)."
        n155 = Obtain Queue(element data type=w344) -> (queue out=w333:refnum<queue>, error out=w343:errorcluster)  [unwired: 4 in, 1 out]
        n156 = Obtain Queue(element data type=w344) -> (queue out=w334:refnum<queue>, error out=w342:errorcluster)  [unwired: 4 in, 1 out]
        n157 = local read "GPIB ADDRESS"() -> (w337:string)
        n158 = Merge Errors(w343, w342) -> (w341:errorcluster)
        n159 = local read "Base Path"() -> (w349:path)
        n160 = vi-ref "GPIB_UART.lvlib:Agilent_GPIB_FSM.vi"() -> (w336:refnum<vi>)
        n161 = Merge Errors(w341, w340) -> (w339:errorcluster)
        n162 = Path To String(path=w349) -> (string=w348:string)
        n163 = Concatenate Strings(w348, "\\labview\\Agilent_GPIB_FSM.vi" ("string")) -> (w346:string)
        n164 = String To Path(string=w346) -> (path=w345:path)
        n165 = Open VI Reference(type specifier VI Refnum (for type only)=w336, vi path=w345, options=128, error in (no error)=w339) -> (vi reference=w335:refnum<vi>, error out=w338:errorcluster)  [unwired: 2 in]
        n166 = call-by-ref "Start Asynchronous Call"(reference=w335, error in=w338, "error in"=w338, "MEAS"=w333, "GPIB"=w337, "commands"=w334) -> (error out=w350:errorcluster)  [unwired: 7 in, 1 out]
      }
      frame "SHUTDOWN" {
        # "Shutdown gracefully."
        n167 = Flush Queue(queue=w354, error in (no error)=w353) -> ()  [unwired: 3 out]
        n168 = flat-sequence {
          tunnel: w360 -> [w367]
          tunnel: w353 -> [w365]
          tunnel: [w364] -> w358
          tunnel: [w363] -> w357
          tunnel: w358 -> [w373]
          tunnel: w357 -> [w371]
          tunnel: [w370] -> w356
          tunnel: [w369] -> w355
          frame #0 {
            n169 = Wait Until Next ms Multiple(millisecond multiple=u32 100) -> ()  [unwired: 1 out]
            n170 = Enqueue Element(queue=w367, element="RESET", error in (no error)=w365) -> (queue out=w364:refnum<queue>, error out=w363:errorcluster)  [unwired: 1 in, 1 out]
          }
          frame #1 {
            n171 = Wait Until Next ms Multiple(millisecond multiple=u32 100) -> ()  [unwired: 1 out]
            n172 = Enqueue Element(queue=w373, element="SHUTDOWN", error in (no error)=w371) -> (queue out=w370:refnum<queue>, error out=w369:errorcluster)  [unwired: 1 in, 1 out]
          }
        }
      }
      frame "ERROR" {
        # "Release (Destroy) Queues"
        n173 = Preview Queue Element(queue=w376, error in (no error)=w378) -> (queue out=w374:refnum<queue>, error out=w382:errorcluster)  [unwired: 1 in, 2 out]
        n174 = Preview Queue Element(queue=w377, error in (no error)=w378) -> (queue out=w375:refnum<queue>, error out=w381:errorcluster)  [unwired: 1 in, 2 out]
        n175 = Merge Errors(w382, w381) -> (w380:errorcluster)
      }
      frame "IDLE", Default {
      }
      frame "READ ERROR" {
        # "Sends a command to the Finite State Machine to clear any error."
        n176 = Enqueue Element(queue=w388, element="READ:ERROR", error in (no error)=w391) -> (queue out=w386:refnum<queue>, error out=w389:errorcluster)  [unwired: 1 in, 1 out]
      }
      frame "RESET" {
        # "Sends a command to the Finite State Machine to reset the power supply to the settings as when it was turned on the first time."
        n177 = Enqueue Element(queue=w393, element="RESET", error in (no error)=w396) -> (queue out=w392:refnum<queue>, error out=w395:errorcluster)  [unwired: 1 in, 1 out]
      }
      frame "VOLTAGE 12" {
        # "Sends a command to the Finite State Machine to output a voltage that can power the air pump."
        n178 = Enqueue Element(queue=w400, element="VOLT 12", error in (no error)=w403) -> (queue out=w398:refnum<queue>, error out=w402:errorcluster)  [unwired: 1 in, 1 out]
      }
      frame "VOLTAGE 0" {
        # "Sends a command to the Finite State Machine to stop outputting a voltage that can power the air pump."
        n179 = Enqueue Element(queue=w406, element="VOLT 0", error in (no error)=w408) -> (queue out=w405:refnum<queue>, error out=w407:errorcluster)  [unwired: 1 in, 1 out]
      }
      frame "RAMP STEP" {
      }
    }
    n180 = Wait Until Next ms Multiple(millisecond multiple=u32 20) -> ()  [unwired: 1 out]
    n181 = call <vilib>:"Clear Errors.vi"("error in (no error)"=w267) -> ("error out"=w268:errorcluster)  [unwired: 5 in, 1 out]
  }
  n182 = while {
    tunnel: w33 -> [w440]
    shift-right: [w438] -> w5
    shift-left: w12 -> [w439]
    tunnel: w28 -> [w437]
    tunnel: [w436] -> w27
    tunnel: [w435] -> w26
    tunnel: w17 -> [w430]
    tunnel: [w425] -> w6
    stop <- w427 stop-if-true
    # "Guard Clause"
    # "PRODUCER LOOP"
    n183 = event shown="[13] \"Save As Button\": Value Change" {
      selector: _ -> [_ _ _ _ _ _ _ _ _ _ _ _ _ _ _ _ _ _ _ _ _]
      dyn-events: _ -> [_ _ _ _ _ _ _ _ _ _ _ _ _ _ _ _ _ _ _ _ _]
      timeout: _ -> [_ _ _ _ _ _ _ _ _ _ _ _ _ _ _ _ _ _ _ _ _]
      tunnel: w440 -> [w462 _ w476 _ _ w490 _ _ _ _ w551 _ _ _ w598 _ w644 w650 _ _ w678]
      tunnel: w439 -> [w460 _ w470 w480 _ w488 w510 w520 w530 w540 w550 w570 w587 _ w600 w629 w642 w648 w654 w668 w675]
      tunnel: [w458 _ w468 w478 _ w485 w509 w518 w528 w538 w547 w569 w579 _ w591 w628 w636 w646 w652 w662 w676] -> w434
      tunnel: [_ _ w472 _ _ w489 _ _ _ _ _ _ _ _ w593 _ w639 w647 _ _ w677] -> w432
      tunnel: w437 -> [_ _ _ _ _ _ w516 w526 w536 w543 w549 _ w589 _ w603 w634 _ _ w660 w673 _]
      tunnel: [_ _ _ _ _ _ w512 w524 w534 w542 _ _ w588 _ w592 _ _ _ w656 w671 _] -> w433
      tunnel: w430 -> [_ _ _ _ _ _ _ _ _ _ w548 _ _ _ w599 _ _ _ _ _ _]
      tunnel: [FALSE FALSE FALSE FALSE FALSE FALSE FALSE FALSE FALSE FALSE FALSE FALSE FALSE FALSE TRUE FALSE FALSE FALSE FALSE FALSE FALSE] -> w428
      tunnel: [_ _ _ _ _ _ _ _ _ _ _ _ _ _ w594 _ _ _ _ _ _] -> w426
      event "BAUD": Value Change {
        # "Baud Rate Value Changed. Use #1 Consumer Loop to update \nthe Serial Connection Finite State Machine (FSM) status. \nThen, go back to idle state (wait for next event to happen).\nAlso write on the datalog that this event has happened (same for every event case)."
        n184 = event-data() -> ()  [unwired: 1 in, 1 out]
        n185 = Enqueue Element(queue=w462, element=startup_FSM."CHANGE BAUD", error in (no error)=w460) -> (error out=w458:errorcluster)  [unwired: 1 in, 2 out]
      }
      event "Knob": Value Change {
        n186 = event-data() -> ("NewVal"=w464:ext)  [unwired: 1 in]
        n187 = Multiply(x=w464, y=ext 1000.0) -> (x*y=→"Output Current [mA]":ext)
      }
      event "SAMP. FREQ. [HZ]": Value Change {
        # "Sampling Frequency Value Changed. Use #1 Consumer Loop to update \nthe Serial Connection Finite State Machine (FSM) status."
        n188 = event-data() -> ()  [unwired: 1 in, 1 out]
        n189 = Enqueue Element(queue=w476, element=startup_FSM."CHANGE SAMP. FREQ.", error in (no error)=w470) -> (queue out=w474:refnum<queue>, error out=w473:errorcluster)  [unwired: 1 in, 1 out]
        n190 = Enqueue Element(queue=w474, element=startup_FSM."IDLE", error in (no error)=w473) -> (queue out=w472:refnum<queue>, error out=w469:errorcluster)  [unwired: 1 in, 1 out]
        n191 = Merge Errors(w469) -> (w468:errorcluster)
      }
      event "Commands": Value Change {
        # "A new command was enqueued via the front panel. The EXTERNAL COMMANDS DECODER Loop decodes\nthe instruction.\nAlso write on the datalog that this event has happened (same for every event case)."
        n192 = event-data() -> ()  [unwired: 1 in, 1 out]
        n193 = local read "commands"() -> (w482:refnum<queue>)
        n194 = Enqueue Element(queue=w482, element="Commands", error in (no error)=w480) -> (error out=w479:errorcluster)  [unwired: 1 in, 2 out]
        n195 = Merge Errors(w479) -> (w478:errorcluster)
      }
      event "GPIB ADDRESS": Value Change {
        # "#TO_BE_IMPLEMENTED"
        n196 = event-data() -> ()  [unwired: 1 in, 6 out]
      }
      event "Connect Button": Value Change {
        # "Connect Button Value Changed. Either Connect or Disconnect from Arduino.\nThis depends on the value (either true or false) of the connect button)."
        n197 = event-data() -> ("NewVal"=w487:bool)  [unwired: 1 in]
        n198 = case shown="False" w487 {
          tunnel: w490 -> [w498 w506]
          tunnel: [w494 w502] -> w486
          tunnel: [w493 w501] -> w489
          tunnel: w488 -> [w491 w499]
          frame False {
            n199 = Enqueue Element(queue=w498, element=startup_FSM."DISCONNECT", error in (no error)=w491) -> (queue out=w496:refnum<queue>, error out=w495:errorcluster)  [unwired: 1 in, 1 out]
            n200 = Enqueue Element(queue=w496, element=startup_FSM."IDLE", error in (no error)=w495) -> (queue out=w493:refnum<queue>, error out=w494:errorcluster)  [unwired: 1 in, 1 out]
          }
          frame True {
            n201 = Enqueue Element(queue=w506, element=startup_FSM."CONNECT", error in (no error)=w499) -> (queue out=w504:refnum<queue>, error out=w503:errorcluster)  [unwired: 1 in, 1 out]
            n202 = Enqueue Element(queue=w504, element=startup_FSM."IDLE", error in (no error)=w503) -> (queue out=w501:refnum<queue>, error out=w502:errorcluster)  [unwired: 1 in, 1 out]
          }
        }
        n203 = Merge Errors(w486) -> (w485:errorcluster)
      }
      event "STEP [mA]": Value Change {
        # "Current Ramp Step Value Changed. Use the #4 Consumer Loop \nto update the Current Ramp Finite  State Machine status."
        n204 = event-data() -> ()  [unwired: 1 in, 1 out]
        n205 = Enqueue Element(queue=w516, element=dc_ps_FSM."RAMP STEP", error in (no error)=w510) -> (queue out=w514:refnum<queue>, error out=w511:errorcluster)  [unwired: 1 in, 1 out]
        n206 = Enqueue Element(queue=w514, element=dc_ps_FSM."IDLE", error in (no error)=w511) -> (queue out=w512:refnum<queue>, error out=w508:errorcluster)  [unwired: 1 in, 1 out]
        n207 = Merge Errors(w508) -> (w509:errorcluster)
      }
      event "OUTPUT CHANNEL": Value Change {
        # "Changed the Power Supply Output Channel (either 25V or 50V)"
        n208 = event-data() -> ()  [unwired: 1 in, 1 out]
        n209 = Enqueue Element(queue=w526, element=dc_ps_FSM."SELECT CH", error in (no error)=w520) -> (queue out=w525:refnum<queue>, error out=w523:errorcluster)  [unwired: 1 in, 1 out]
        n210 = Enqueue Element(queue=w525, element=dc_ps_FSM."IDLE", error in (no error)=w523) -> (queue out=w524:refnum<queue>, error out=w519:errorcluster)  [unwired: 1 in, 1 out]
        n211 = Merge Errors(w519) -> (w518:errorcluster)
      }
      event "READ ERROR": Value Change {
        # "When a Power Supply Error (like requiring to output 30V using a 25V output channel) it is required to Read (clear) the error to continue to use the instrument."
        n212 = event-data() -> ()  [unwired: 1 in, 1 out]
        n213 = Enqueue Element(queue=w536, element=dc_ps_FSM."READ ERROR", error in (no error)=w530) -> (queue out=w535:refnum<queue>, error out=w533:errorcluster)  [unwired: 1 in, 1 out]
        n214 = Enqueue Element(queue=w535, element=dc_ps_FSM."IDLE", error in (no error)=w533) -> (queue out=w534:refnum<queue>, error out=w529:errorcluster)  [unwired: 1 in, 1 out]
        n215 = Merge Errors(w529) -> (w528:errorcluster)
      }
      event "RESET & CLEAR": Value Change {
        n216 = event-data() -> ()  [unwired: 1 in, 1 out]
        n217 = Enqueue Element(queue=w543, element=dc_ps_FSM."RESET", error in (no error)=w540) -> (queue out=w542:refnum<queue>, error out=w539:errorcluster)  [unwired: 1 in, 1 out]
        n218 = Merge Errors(w539) -> (w538:errorcluster)
      }
      event "CURRENT RAMP": Value Change {
        n219 = event-data() -> ("NewVal"=w552:bool)  [unwired: 1 in]
        n220 = case shown="True" w552 {
          tunnel: w551 -> [_ _]
          tunnel: w550 -> [_ w566]
          tunnel: [_ w562] -> w545
          tunnel: w549 -> [_ w568]
          tunnel: w548 -> [w555 w558]
          tunnel: [w554 w561] -> w546
          frame False {
            # "Change the state in the \nCurrent Ramp FSM.\nDisable the ramp."
            n221 = Enqueue Element(queue=w555, element=current_ramp_FSM."RAMP DISABLE") -> (error out=w554:errorcluster)  [unwired: 2 in, 2 out]
          }
          frame True {
            # "Set the output to 0mA."
            # "Change the state of the Current Ramp\nFinite State Machine. Used to start the Current Ramp."
            n222 = property on="Knob" class="Knob (strict)"("Val(Sgnl)"=0.0 ("Knob")) -> ()  [unwired: 2 in, 2 out]
            n223 = Flush Queue(queue=w558) -> (queue out=w557:refnum<queue>, error out=w556:errorcluster)  [unwired: 1 in, 1 out]
            n224 = Enqueue Element(queue=w568, element=dc_ps_FSM."OUT CURR", error in (no error)=w566) -> (queue out=w565:refnum<queue>, error out=w564:errorcluster)  [unwired: 1 in, 1 out]
            n225 = Enqueue Element(queue=w557, element=current_ramp_FSM."RAMP ENABLE", error in (no error)=w556) -> (error out=w561:errorcluster)  [unwired: 1 in, 2 out]
            n226 = Enqueue Element(queue=w565, element=dc_ps_FSM."IDLE", error in (no error)=w564) -> (error out=w562:errorcluster)  [unwired: 1 in, 2 out]
          }
        }
        n227 = Merge Errors(w546, w545) -> (w547:errorcluster)
      }
      event "Next": Value Change {
        # "If the Current Ramp has been enabled, \nthen, when the next button is pressed\neither two things could happen.\nThe output current is increased (Ramp Up State)\nor decreased (Ramp Down State).\nSignal that a transition to the next state is required."
        n228 = event-data() -> ()  [unwired: 1 in, 1 out]
        n229 = local read "CURRENT RAMP"() -> (w571:bool)
        n230 = case shown="True" w571 {
          tunnel: [w573 w574] -> w569
          tunnel: w570 -> [w573 w575]
          frame False {
          }
          frame True {
            n231 = property on="Next Current Ramp State" class="Bool (strict)"(error in=w575, "Val(Sgnl)"=TRUE ("Value (Signaling)")) -> (error out=w574:errorcluster)  [unwired: 1 in, 1 out]
          }
        }
      }
      event "VOLTAGE": Value Change {
        # "When \"Voltage\" Value Changes then\nthe power supply output voltage is either 0V (false)\nor 12V (true)"
        n232 = event-data() -> ("NewVal"=w583:bool)  [unwired: 1 in]
        n233 = Select(t=dc_ps_FSM."VOLTAGE 12" ("element"), s=w583, f=dc_ps_FSM."VOLTAGE 0") -> (s? t:f=w580:T2)
        n234 = Enqueue Element(queue=w589, element=w580, error in (no error)=w587) -> (queue out=w586:refnum<queue>, error out=w585:errorcluster)  [unwired: 1 in, 1 out]
        n235 = Enqueue Element(queue=w586, element=dc_ps_FSM."IDLE", error in (no error)=w585) -> (queue out=w588:refnum<queue>, error out=w578:errorcluster)  [unwired: 1 in, 1 out]
        n236 = Merge Errors(w578) -> (w579:errorcluster)
      }
      event "Save As Button": Value Change {
        # "#TO_BE_IMPLEMENTED"
        n237 = event-data() -> ()  [unwired: 1 in, 1 out]
      }
      event "Stop Button": Value Change {
        n238 = event-data() -> ()  [unwired: 1 in, 1 out]
        n239 = flat-sequence {
          tunnel: w603 -> [w612]
          tunnel: [w612] -> w601
          tunnel: w600 -> [w611]
          tunnel: w599 -> [w610]
          tunnel: w598 -> [w608]
          tunnel: [w608] -> w597
          tunnel: [w607] -> w596
          tunnel: [w606] -> w594
          tunnel: [w619] -> w602
          tunnel: w601 -> [w619]
          tunnel: w597 -> [w618]
          tunnel: w596 -> [w617]
          tunnel: [w616] -> w595
          tunnel: [w614] -> w593
          tunnel: w602 -> [w625]
          tunnel: w595 -> [w623]
          tunnel: [w622] -> w592
          tunnel: [w621] -> w591
          frame #0 {
            n240 = Enqueue Element(queue=w610, element=current_ramp_FSM."SHUTDOWN", error in (no error)=w611) -> (queue out=w606:refnum<queue>, error out=w607:errorcluster)  [unwired: 1 in, 1 out]
            n241 = Wait Until Next ms Multiple(millisecond multiple=u32 20) -> ()  [unwired: 1 out]
          }
          frame #1 {
            n242 = Wait Until Next ms Multiple(millisecond multiple=u32 20) -> ()  [unwired: 1 out]
            n243 = Enqueue Element(queue=w618, element=startup_FSM."SHUTDOWN", error in (no error)=w617) -> (queue out=w614:refnum<queue>, error out=w616:errorcluster)  [unwired: 1 in, 1 out]
          }
          frame #2 {
            n244 = Enqueue Element(queue=w625, element=dc_ps_FSM."SHUTDOWN", error in (no error)=w623) -> (queue out=w622:refnum<queue>, error out=w621:errorcluster)  [unwired: 1 in, 1 out]
            n245 = Wait Until Next ms Multiple(millisecond multiple=u32 20) -> ()  [unwired: 1 out]
          }
        }
      }
      event "CURRENT LIMIT [mA]": Value Change {
        # "Output Current Limit Value Changed. Used by the Current Ramp\nFinite State Machine."
        n246 = event-data() -> ()  [unwired: 1 in, 2 out]
        n247 = Enqueue Element(queue=w634, element=dc_ps_FSM."LIMITS", error in (no error)=w629) -> (queue out=w633:refnum<queue>, error out=w630:errorcluster)  [unwired: 1 in, 1 out]
        n248 = Enqueue Element(queue=w633, element=dc_ps_FSM."IDLE", error in (no error)=w630) -> (error out=w627:errorcluster)  [unwired: 1 in, 2 out]
        n249 = Merge Errors(w627) -> (w628:errorcluster)
      }
      event "Clear Buffer": Value Change {
        # "When this button is pushed than the buffer\nwhere it is stored the serial data (digital flow sensor measurements)\nis flushed (cleared). This is useful to read the latest data."
        n250 = event-data() -> ()  [unwired: 1 in, 1 out]
        n251 = Enqueue Element(queue=w644, element=startup_FSM."CLEAR BUFF", error in (no error)=w642) -> (queue out=w641:refnum<queue>, error out=w640:errorcluster)  [unwired: 1 in, 1 out]
        n252 = Enqueue Element(queue=w641, element=startup_FSM."IDLE", error in (no error)=w640) -> (queue out=w639:refnum<queue>, error out=w637:errorcluster)  [unwired: 1 in, 1 out]
        n253 = Merge Errors(w637) -> (w636:errorcluster)
      }
      event "SERIAL PORT": Value Change {
        n254 = event-data() -> ()  [unwired: 1 in, 1 out]
        n255 = Enqueue Element At Opposite End(queue=w650, element=startup_FSM."CHANGE PORT", error in (no error)=w648) -> (queue out=w647:refnum<queue>, error out=w646:errorcluster)  [unwired: 1 in, 1 out]
      }
      event "ADJUST": Value Change {
        # "The knob does not change the output current directly.\nTo effectively change it the Adjust button has to be pressed."
        n256 = event-data() -> ()  [unwired: 1 in, 1 out]
        n257 = Enqueue Element(queue=w660, element=dc_ps_FSM."OUT CURR", error in (no error)=w654) -> (queue out=w659:refnum<queue>, error out=w658:errorcluster)  [unwired: 1 in, 1 out]
        n258 = Enqueue Element(queue=w659, element=dc_ps_FSM."IDLE", error in (no error)=w658) -> (queue out=w656:refnum<queue>, error out=w653:errorcluster)  [unwired: 1 in, 1 out]
        n259 = Merge Errors(w653) -> (w652:errorcluster)
      }
      event "POWER SUPPLY OUTPUT": Value Change {
        # "When the POWER SUPPLY OUTPUT is pressed\nit either enables or disables the output line of\nthe power supply"
        n260 = event-data() -> ("NewVal"=w667:bool)  [unwired: 1 in]
        n261 = Select(t=dc_ps_FSM."OUTPUT ON" ("element"), s=w667, f=dc_ps_FSM."OUTPUT OFF") -> (s? t:f=w664:T2)
        n262 = Enqueue Element(queue=w673, element=w664, error in (no error)=w668) -> (queue out=w672:refnum<queue>, error out=w670:errorcluster)  [unwired: 1 in, 1 out]
        n263 = Enqueue Element(queue=w672, element=dc_ps_FSM."IDLE", error in (no error)=w670) -> (queue out=w671:refnum<queue>, error out=w663:errorcluster)  [unwired: 1 in, 1 out]
        n264 = Merge Errors(w663) -> (w662:errorcluster)
      }
      event "Read Button": Value Change {
        # "When the true, read from the serial data queue.\nWhen false stop reading."
        n265 = event-data() -> ("NewVal"=w679:bool)  [unwired: 1 in]
        n266 = case shown="True" w679 {
          tunnel: w678 -> [w684 w689]
          tunnel: [w683 w688] -> w677
          tunnel: w675 -> [w682 w685]
          tunnel: [w681 w687] -> w676
          frame False {
            n267 = Enqueue Element(queue=w684, element=startup_FSM."IDLE", error in (no error)=w682) -> (queue out=w683:refnum<queue>, error out=w681:errorcluster)  [unwired: 1 in, 1 out]
          }
          frame True {
            n268 = Enqueue Element(queue=w689, element=startup_FSM."READ", error in (no error)=w685) -> (queue out=w688:refnum<queue>, error out=w687:errorcluster)  [unwired: 1 in, 1 out]
          }
        }
      }
    }
    n269 = Wait Until Next ms Multiple(millisecond multiple=u32 10) -> ()  [unwired: 1 out]
    n270 = case shown="No Error" w434 {
      selector: w434 -> [w444 w455]
      tunnel: [w445 w448] -> w435
      tunnel: w432 -> [w445 w456]
      tunnel: [w444 w450] -> w438
      tunnel: w433 -> [w443 w457]
      tunnel: [w443 w449] -> w436
      tunnel: [FALSE FALSE] -> w429
      tunnel: w426 -> [w441 w446]
      tunnel: [w441 w446] -> w425
      frame No Error {
      }
      frame Error {
        n271 = Enqueue Element(queue=w457, element=dc_ps_FSM."ERROR", error in (no error)=w455) -> (queue out=w449:refnum<queue>, error out=w452:errorcluster)  [unwired: 1 in, 1 out]
        n272 = Enqueue Element(queue=w456, element=startup_FSM."ERROR", error in (no error)=w455) -> (queue out=w448:refnum<queue>, error out=w451:errorcluster)  [unwired: 1 in, 1 out]
        n273 = Merge Errors(w452, w451) -> (w450:errorcluster)
      }
    }
    n274 = Or(x=w429, y=w428) -> (x .or. y?=w427:bool)
  }
  n275 = while {
    tunnel: w33 -> [w707]
    shift-right: [w690] -> w23
    shift-left: w7 -> [w708]
    tunnel: [w701] -> w20
    shift-right: [w698] -> _
    shift-left: dbl[] [] -> [w700]
    tunnel: "measurements" -> [w699]
    shift-right: [w697] -> _
    shift-left: _ -> [w695]
    shift-right: [w696] -> _
    shift-left: _ -> [w694]
    stop <- w703 stop-if-true
    # "#1 CONSUMER LOOP : SERIAL CONNECTION FSM"
    n276 = case shown="No Error" w708 {
      selector: w708 -> [w825 w831]
      tunnel: w707 -> [w826 w830]
      tunnel: [w824 w831] -> w706
      tunnel: [w823 w830] -> w705
      tunnel: [w822 startup_FSM."ERROR" ("element")] -> w704
      tunnel: [w821 w828] -> w692
      tunnel: w695 -> [w821 w828]
      tunnel: [w820 w827] -> w693
      tunnel: w694 -> [w820 w827]
      frame No Error {
        # "Guard Clause"
        n277 = Dequeue Element(queue=w826, error in (no error)=w825) -> (queue out=w823:refnum<queue>, element=w822:T3, error out=w824:errorcluster)  [unwired: 1 in, 1 out]
      }
      frame Error {
        # "Guard Clause"
      }
    }
    n278 = case shown="\"INIT\"" w704 {
      tunnel: w706 -> [w718 w734 w757 w763 w776 w782 w796 w803 w806 w813 w819]
      tunnel: w705 -> [_ w731 _ _ _ w785 _ _ _ _ _]
      tunnel: [w727 w739 w752 w762 w775 _ w795 w801 w807 w813 w818] -> w691
      tunnel: [FALSE TRUE _ _ _ _ _ _ FALSE _ _] -> w703
      tunnel: [w728 _ _ _ _ _ _ _ _ _ _] -> w701
      tunnel: w700 -> [_ _ _ _ _ w784 _ _ _ _ _]
      tunnel: w699 -> [_ _ _ _ _ w786 _ _ _ _ _]
      tunnel: [_ _ _ _ _ w780 _ _ _ _ _] -> w698
      tunnel: [w713 w737 w751 w758 w772 w778 w792 w798 w804 w812 w815] -> w697
      tunnel: [w712 w738 w753 w759 w773 w777 w793 w799 w805 w811 w814] -> w696
      tunnel: w693 -> [_ w735 w754 w760 w774 w777 w794 w800 w809 w811 w814]
      tunnel: w692 -> [_ w737 w751 w758 w772 w779 w792 w798 w804 w812 w816]
      frame "INIT" {
        w715 = ""
        # "reset is the initial state"
        # "this is a reference\nlike a pointer in C"
        # "start the subVI"
        # "x80 means \"call and forget\""
        # "This is the initialization state.\nThe SubVI is called #asynchronously (call and forget).\nThis means that we do not wait for the sub-program to finish its execution\n(infact the subVI enters a while loop until this program is shutdown)."
        n279 = local read "Base Path"() -> (w726:path)
        n280 = vi-ref "GPIB_UART.lvlib:Arduino_Serial_FSM.vi"() -> (w709:refnum<vi>)
        n281 = Obtain Queue(element data type=w715) -> (queue out=w713:refnum<queue>, error out=w719:errorcluster)  [unwired: 4 in, 1 out]
        n282 = Obtain Queue(element data type=w715) -> (queue out=w722:refnum<queue>, error out=w721:errorcluster)  [unwired: 4 in, 1 out]
        n283 = Enqueue Element(queue=w722, element="RESET", error in (no error)=w721) -> (queue out=w712:refnum<queue>, error out=w720:errorcluster)  [unwired: 1 in, 1 out]
        n284 = Path To String(path=w726) -> (string=w725:string)
        n285 = Concatenate Strings(w725, "\\labview\\Arduino_Serial_FSM.vi" ("string")) -> (w724:string)
        n286 = String To Path(string=w724) -> (path=w723:path)
        n287 = Open VI Reference(type specifier VI Refnum (for type only)=w709, vi path=w723, options=128, error in (no error)=w718) -> (vi reference=w710:refnum<vi>, error out=w717:errorcluster)  [unwired: 2 in]
        n288 = Merge Errors(w717, w719, w720) -> (w716:errorcluster)
        n289 = call-by-ref "Start Asynchronous Call"(reference=w710, error in=w716, "commands_q"=w712, "sensor_data_q"=w713, 11:"error in (no error)"=w716) -> (reference out=w728:refnum<vi>, error out=w727:errorcluster)  [unwired: 12 in, 1 out]
      }
      frame "SHUTDOWN" {
        n290 = flat-sequence {
          tunnel: w734 -> [w741]
          tunnel: w735 -> [w743]
          tunnel: [w743] -> w733
          tunnel: [w741] -> w732
          tunnel: w731 -> [w742]
          tunnel: [w749] -> w739
          tunnel: [w747] -> w738
          tunnel: w733 -> [w746]
          tunnel: w732 -> [w745]
          frame #0 {
            n291 = Flush Queue(queue=w742, error in (no error)=w741) -> ()  [unwired: 3 out]
            n292 = Wait Until Next ms Multiple(millisecond multiple=u32 100) -> ()  [unwired: 1 out]
          }
          frame #1 {
            n293 = Wait Until Next ms Multiple(millisecond multiple=u32 100) -> ()  [unwired: 1 out]
            n294 = Enqueue Element(queue=w746, element="SHUTDOWN", error in (no error)=w745) -> (queue out=w747:refnum<queue>, error out=w749:errorcluster)  [unwired: 1 in, 1 out]
          }
        }
      }
      frame "CHANGE BAUD" {
        # "Sends a command to the Finite State Machine.\nThis does not alter the current connection.\nDisconnect and Connect Again to see a difference."
        n295 = local read "BAUD"() -> (w750:string)
        n296 = Concatenate Strings("SET:BAUD ", w750) -> (w755:string)
        n297 = Enqueue Element(queue=w754, element=w755, error in (no error)=w757) -> (queue out=w753:refnum<queue>, error out=w752:errorcluster)  [unwired: 1 in, 1 out]
      }
      frame "CHANGE SAMP. FREQ." {
        # "Sends a command to the Finite State Machine.\nThis alters directly the current connection.\nThe Arduino Board will output measurements more quicly or more slowly."
        n298 = Number To Fractional String(number="SAMP. FREQ. [HZ]", precision (6)=i16 2) -> (F-format string=w765:string)  [unwired: 2 in]
        n299 = Concatenate Strings("SF " ("string"), w765) -> (w764:string)
        n300 = Enqueue Element(queue=w760, element=w764, error in (no error)=w763) -> (queue out=w759:refnum<queue>, error out=w762:errorcluster)  [unwired: 1 in, 1 out]
      }
      frame "CHANGE PORT" {
        # "Sends a command to the Finite State Machine.\nThis does not alter the current connection.\nDisconnect and Connect Again to see a difference."
        n301 = call <vilib>:"Space Constant.vi"() -> ("String"=w768:string)
        n302 = local read "SERIAL PORT"() -> (w770:string)
        n303 = call "conc_state_args.vi"("State"="SET:PORT" ("element"), "DELIMITER (:)"=w768, "Args"=w770) -> ("state_and_args"=w769:string)  [unwired: 12 in]
        n304 = Enqueue Element(queue=w774, element=w769, error in (no error)=w776) -> (queue out=w773:refnum<queue>, error out=w775:errorcluster)  [unwired: 1 in, 1 out]
      }
      frame "READ" {
        # "Enqueue data in the Measurements Queue read by the MainVI."
        # "Continue Reading by feeding this state continuosly."
        # "FSM"
        n305 = local read "Read Button"() -> (w790:bool)
        n306 = Dequeue Element(queue=w779) -> (queue out=w778:refnum<queue>, element=w791:string)  [unwired: 2 in, 2 out]
        n307 = Select(t=startup_FSM."READ" ("element"), s=w790, f=startup_FSM."IDLE") -> (s? t:f=w789:T3)
        n308 = Enqueue Element(queue=w785, element=w789, error in (no error)=w782) -> ()  [unwired: 1 in, 3 out]
        n309 = Enqueue Element(queue=w786, element=w791, error in (no error)=w782) -> ()  [unwired: 1 in, 3 out]
        n310 = Fract/Exp String To Number(string=w791) -> (number=w783:dbl)  [unwired: 3 in, 1 out]
        "flow meas" <- w783
        n311 = Build Array (concatenate) "Build Array"(w784, w783) -> (w780:dbl[])
        "Arduino UNO Controls" <- w780
        n312 = Array Size(array=w780) -> (size(s)=→"SAMPLE  COUNT":i32)
      }
      frame "DISCONNECT" {
        # "Sends a command to the Finite State Machine to disconnect from the Arduino Board."
        n313 = Enqueue Element(queue=w794, element="DISCONNECT", error in (no error)=w796) -> (queue out=w793:refnum<queue>, error out=w795:errorcluster)  [unwired: 1 in, 1 out]
      }
      frame "CONNECT" {
        # "Sends a command to the Finite State Machine to connect from the Arduino Board using the  COM port and Baud Rate Selected"
        n314 = Enqueue Element(queue=w800, element="CONNECT", error in (no error)=w803) -> (queue out=w799:refnum<queue>, error out=w801:errorcluster)  [unwired: 1 in, 1 out]
      }
      frame "ERROR" {
        # "Shutdown gracefully."
        n315 = Enqueue Element(queue=w809, element="SHUTDOWN", error in (no error)=w806) -> (queue out=w805:refnum<queue>, error out=w807:errorcluster)  [unwired: 1 in, 1 out]
      }
      frame "IDLE", Default {
        # "wait for next action by entering the next loop iteration\n and by stopping at dequeue next element\nin the guard clause"
        # "do nothing."
      }
      frame "CLEAR BUFF" {
        # "basically clear the graph on the front panel, reset the sample count to zero and flush the queue\nthat stores past measurements already transferred."
        n316 = invoke on="Arduino UNO Controls" class="WFGraph (strict)" method="Reinit To Default"() -> ()  [unwired: 3 in, 3 out]
        n317 = local write "SAMPLE  COUNT"(0.0) -> ()
        n318 = Flush Queue(queue=w816, error in (no error)=w819) -> (queue out=w815:refnum<queue>, error out=w818:errorcluster)  [unwired: 1 out]
      }
    }
    n319 = Wait Until Next ms Multiple(millisecond multiple=u32 20) -> ()  [unwired: 1 out]
    n320 = call <vilib>:"Clear Errors.vi"("error in (no error)"=w691) -> ("error out"=w690:errorcluster)  [unwired: 5 in, 1 out]
  }
  n321 = Close Reference(reference=w20) -> ()  [unwired: 1 in, 1 out]
  n322 = Release Queue(queue=w6, error in (no error)=w5) -> (error out=w4:errorcluster)  [unwired: 1 in, 2 out]
  n323 = Release Queue(queue=w27, error in (no error)=w5) -> (error out=w25:errorcluster)  [unwired: 1 in, 2 out]
  n324 = Release Queue(queue=w26, error in (no error)=w5) -> (error out=w24:errorcluster)  [unwired: 1 in, 2 out]
  n325 = Merge Errors(w4, w25, w24, w23, w22, w13) -> (w21:errorcluster)
  n326 = call <vilib>:"Simple Error Handler.vi"("error in (no error)"=w21) -> ()  [unwired: 4 in, 5 out]
